vi "AutoThresholdLocalization-2.vi"(6 "[IN] Autothreshold Images \nInstead Of Generated U8":bool, 7 "[IN] Method":i32(ring) items=["clustering", "entropy", "metric", "moments", "inter-class variance"], 8 "error IN":errorcluster, 10 "[IN] Binarized Image":T3, 11 "[IN] Source Image":T3) -> (0 "error OUT":errorcluster, 2 "[OUT] X,Y Coordinates":dbl[](array[numeric]))   [LabVIEW 2020]
uses:
  <vilib>/vision/Image Controls.llb/IMAQ Image.ctl
  <vilib>/vision/NI_Vision_Development_Module.lvlib
panel:
  in  "Selection Values":T2(array[cluster])=[{"Measurement Parameter"=22, "Range Lower Value"=10.0, "Range Upper Value"=800.0, "Range"=FALSE, "Measurement Type"=FALSE}] {"Measurement Parameter" items=["Center of Mass X", "Center of Mass Y", "First Pixel X", "First Pixel Y", "Bounding Rect Left", "Bounding Rect Top", "Bounding Rect Right", "Bounding Rect Bottom", "Max Feret Diameter Start X", "Max Feret Diameter Start Y", "Max Feret Diameter End X", "Max Feret Diameter End Y", "Max Horiz. Segment Length Left", "Max Horiz. Segment Length Right", "Max Horiz. Segment Length Row", "-", "Bounding Rect Width", "Bounding Rect Height", "Bounding Rect Diagonal", "Perimeter", "Convex Hull Perimeter", "Holes' Perimeter", "Max Feret Diameter", "Equivalent Ellipse Major Axis", "Equivalent Ellipse Minor Axis", "Equivalent Ellipse Minor Axis (Feret)", "Equivalent Rect Long Side", "Equivalent Rect Short Side", "Equivalent Rect Diagonal", "Equivalent Rect Short Side (Feret)", "Average Horiz. Segment Length", "Average Vert. Segment Length", "Hydraulic Radius", "Waddel Disk Diameter", "-", "Area", "Holes' Area", "Particle & Holes' Area", "Convex Hull Area", "Image Area", "-", "Number of Holes", "Number of Horiz. Segments", "Number of Vert. Segments", "-", "Orientation", "Max Feret Diameter Orientation", "-", "% Area/Image Area", "% Area/(Particle & Holes' Area)", "Ratio of Equivalent Ellipse Axes", "Ratio of Equivalent Rect Sides", "-", "Elongation Factor", "Compactness Factor", "Heywood Circularity Factor", "Type Factor", "-", "Sum X", "Sum Y", "Sum XX", "Sum XY", "Sum YY", "Sum XXX", "Sum XXY", "Sum XYY", "Sum YYY", "-", "Moment of Inertia XX", "Moment of Inertia XY", "Moment of Inertia YY", "Moment of Inertia XXX", "Moment of Inertia XXY", "Moment of Inertia XYY", "Moment of Inertia YYY", "Norm. Moment of Inertia XX", "Norm. Moment of Inertia XY", "Norm. Moment of Inertia YY", "Norm. Moment of Inertia XXX", "Norm. Moment of Inertia XXY", "Norm. Moment of Inertia XYY", "Norm. Moment of Inertia YYY", "Hu Moment 1", "Hu Moment 2", "Hu Moment 3", "Hu Moment 4", "Hu Moment 5", "Hu Moment 6", "Hu Moment 7"]}
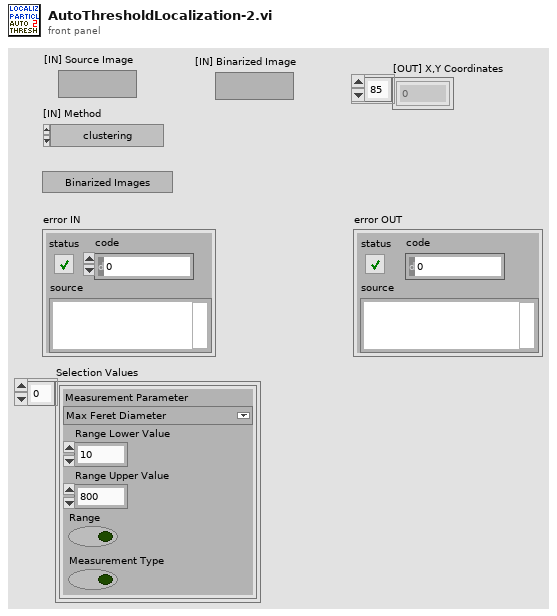
[diagram p1: front panel]
types:
  T1 = typedef "Particle Parameters" = i32
  T2 = cluster{"Measurement Parameter":T1, "Range Lower Value":dbl, "Range Upper Value":dbl, "Range":bool, "Measurement Type":bool}[]
  T3 = typedef "IMAQ Image.ctl" = refnum<image>
  T4 = typedef "Image Type" = u32
  T5 = cluster{"Area":dbl, "Number of Holes":dbl, "Bounding Rect":cluster{"Left":dbl, "Top":dbl, "Right":dbl, "Bottom":dbl}, "Center of Mass":cluster{"X":dbl, "Y":dbl}, "Orientation":dbl, "Dimensions":cluster{"Width":dbl, "Height":dbl}}[]
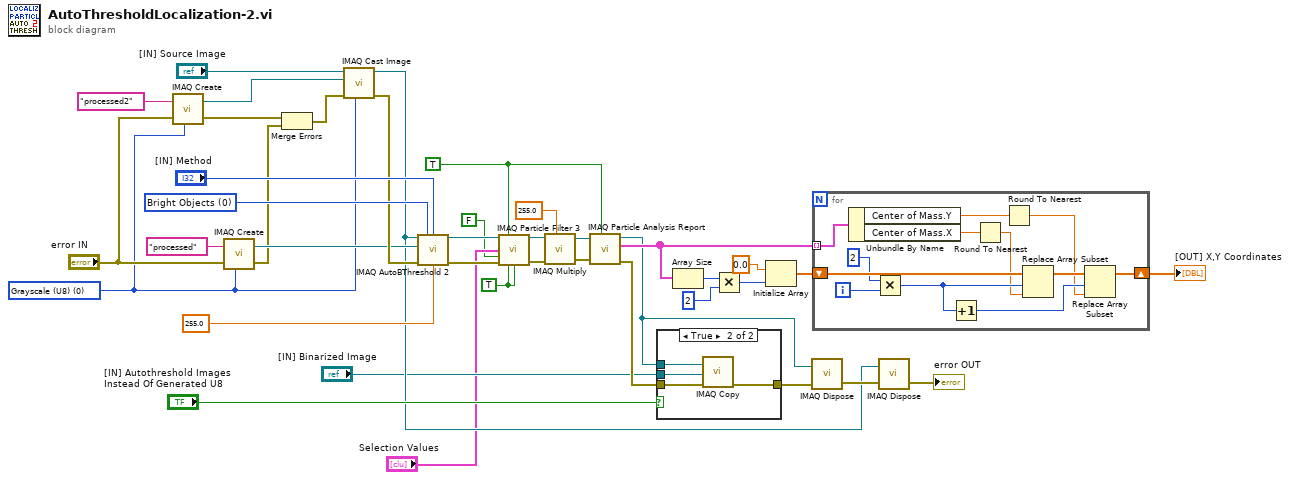
[diagram p0: block diagram]
diagram:
  w6 = TRUE ("Connectivity 4/8 (8)")
  w9 = TRUE ("Connectivity 4/8 (8)")
  w39 = u32 0 items=["Bright Objects", "Dark Objects"] ("Look For (Bright Objects)")
  w19 = T4 0 items=["Grayscale (U8)", "Grayscale (I16)", "Grayscale (SGL)", "Complex (CSG)", "RGB (U32)", "HSL (U32)", "RGB (U64)", "Grayscale (U16)"] ("Image Type")
  n1 = call "IMAQ Create"("Image Name"="processed2", "Image Type"=w19, "error in (no error)"="error IN") -> ("New Image"=w20:T3, "error out"=w18:errorcluster)  [unwired: 2 in]
  n2 = call "IMAQ Create"("Image Name"="processed", "Image Type"=w19, "error in (no error)"="error IN") -> ("New Image"=w23:T3, "error out"=w17:errorcluster)  [unwired: 2 in]
  n3 = Merge Errors(w18, w17) -> (w16:errorcluster)
  n4 = call "IMAQ Cast Image"("Image Type"=w19, "error in (no error)"=w16, "Image Dst"=w20, "Image Src"="[IN] Source Image") -> ("error out"=w24:errorcluster, "Image Dst Out"=w14:T3)  [unwired: 6 in]
  n5 = call "IMAQ AutoBThreshold 2"("Image Src"=w14, "Look For (Bright Objects)"=w39, "Method (clustering)"="[IN] Method", "Image Dst"=w23, "error in (no error)"=w24, "Replace Value (1)"=sgl 255.0) -> ("Image Dst Out"=w10:T3, "error out"=w11:errorcluster)  [unwired: 7 in, 1 out]
  n6 = call "IMAQ Particle Filter 3"("Image Src"=w10, "Connectivity 4/8 (8)"=w9, "Selection Values"="Selection Values", "Keep/Remove Particles (F)"=FALSE, "error in (no error)"=w11, "Reject Border? (F)"=w6, "Fill Holes? (F)"=w6) -> ("Image Dst Out"=w4:T3, "error out"=w5:errorcluster)  [unwired: 6 in, 1 out]
  n7 = call "IMAQ Multiply"("Image Src A"=w4, "Constant"=255.0, "error in (no error)"=w5) -> ("Image Dst Out"=w3:T3, "error out"=w2:errorcluster)  [unwired: 4 in]
  n8 = call "IMAQ Particle Analysis Report"("Connectivity 4/8 (8)"=w9, "error in (no error)"=w2, "Image"=w3) -> ("error out"=w28:errorcluster, "Particle Reports (Pixels)"=w35:T5, "Image Out (duplicate)"=w26:T3)  [unwired: 3 in, 3 out]
  n9 = case shown="True" "[IN] Autothreshold Images \nInstead Of Generated U8" {
    tunnel: w26 -> [_ w45]
    tunnel: w28 -> [w41 w44]
    tunnel: [w41 w43] -> w27
    tunnel: "[IN] Binarized Image" -> [_ w42]
    frame False {
    }
    frame True {
      n10 = call "IMAQ Copy"("error in (no error)"=w44, "Image Dst"=w42, "Image Src"=w45) -> ("error out"=w43:errorcluster)  [unwired: 3 in, 1 out]
    }
  }
  n11 = Array Size(array=w35) -> (size(s)=w34:i32)
  n12 = Multiply(x=w34, y=2) -> (x*y=w32:i32)
  n13 = Initialize Array(0.0 ("element"), w32) -> (w31:dbl[])
  n14 = call "IMAQ Dispose"("Image"=w26, "error in (no error)"=w27) -> ("error out"=w15:errorcluster)  [unwired: 4 in]
  n15 = for {
    tunnel: w35 -> [w57] mode=indexing
    shift-right: [w50] -> w30
    shift-left: w31 -> [w56]
    i -> [w55]
    n16 = Unbundle By Name(w57) -> ("Center of Mass.Y"=w49:dbl, "Center of Mass.X"=w48:dbl)
    n17 = Multiply(x=2 ("y"), y=w55) -> (x*y=w53:i32)
    n18 = Increment(x=w53) -> (x+1=w51:i32)
    n19 = Round To Nearest(number=w48) -> (nearest integer value=w47:dbl)
    n20 = Round To Nearest(number=w49) -> (nearest integer value=w46:dbl)
    n21 = Replace Array Subset(array=w56, new element=w47, index=w53) -> (w52:dbl[])
    n22 = Replace Array Subset(array=w52, new element=w46, index=w51) -> (w50:dbl[])
  }
  "[OUT] X,Y Coordinates" <- w30
  n23 = call "IMAQ Dispose"("Image"=w14, "error in (no error)"=w15) -> ("error out"=→"error OUT":errorcluster)  [unwired: 4 in]
